vi "Read Lines From File Contrario_mio.vi"(2 "convert eol? (no:F)":bool, 3 "file path (dialog if empty)":path, 4 "number of lines (all:-1)":i32=-1, 8 "start of read offset (chars.:0)":i32, 9 "[max characters per line]  (no limit:0)":i32) -> (0 "new file path (Not A Path if cancelled)":path, 1 "line string":string, 5 "mark after read (chars.)":i32, 6 "EOF?":bool)   [LabVIEW 2010]
doc: "Reads a specified number of lines from a byte stream file beginning at a specified character offset. The VI opens the file before reading from it and closes it afterwards."
uses:
  <vilib>/Utility/error.llb/DialogType.ctl
panel:
  out "Numeric":i32
  in  "prompt":string="Choose file to read."
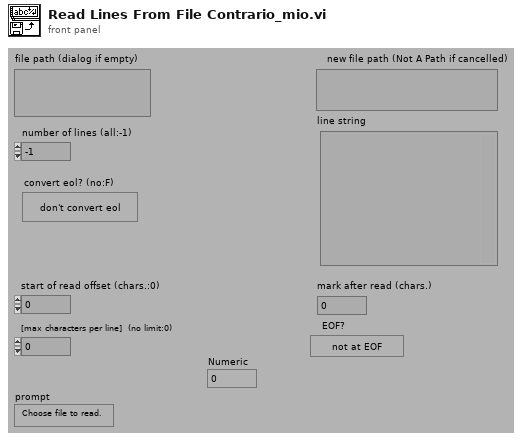
[diagram p1: front panel]
types:
  T1 = typedef "DialogType.ctl" = u16
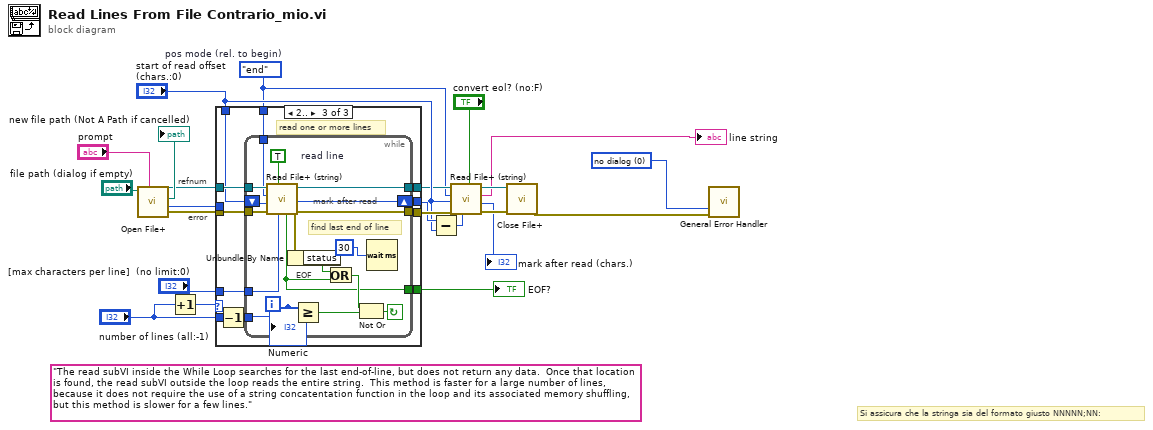
[diagram p0: block diagram]
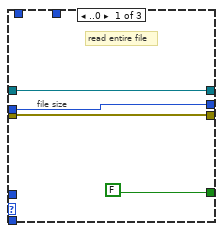
[diagram p2: hidden frame]
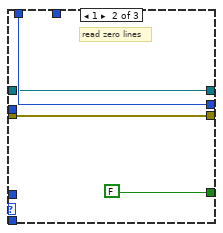
[diagram p3: hidden frame]
diagram:
  w1 = T1 0 items=["no dialog", "OK message", "continue or stop message", "OK message + warnings", "continue/stop + warnings"] ("type of dialog (OK msg:1)")
  w4 = enum16{"start", "end", "current"}."end"  # pos mode (rel. to begin)
  (unwired) "The read subVI inside the While Loop searches for the last end-of-line, but does not return any data.  Once that location is found, the read subVI outside the loop reads the entire string.  This method is faster for a large number of lines, because it does not require the use of a string concatentation function in the loop and its associated memory shuffling, but this method is slower for a few lines."
  # "Si assicura che la stringa sia del formato giusto NNNNN;NN:"
  # "error"
  # "refnum"
  n1 = call <vilib>:"Open File+.vi"("prompt"="prompt", "file path (\" \")"="file path (dialog if empty)") -> ("error out"=w11:errorcluster, "file size (bytes)"=w8:i32, "file path"=→"new file path (Not A Path if cancelled)":path, "refnum"=w10:refnum<file>)  [unwired: 6 in]
  n2 = Increment(x="number of lines (all:-1)") -> (x+1=w13:i32)
  n3 = case shown="2.." w13 {
    tunnel: [w27 w30 w42] -> w15
    tunnel: [w26 w31 w41] -> w14
    tunnel: "number of lines (all:-1)" -> [_ _ w40]
    tunnel: "[max characters per line]  (no limit:0)" -> [_ _ w39]
    tunnel: w11 -> [w27 w30 w38]
    tunnel: w10 -> [w25 w29 w37]
    tunnel: "start of read offset (chars.:0)" -> [_ w31 w36]
    tunnel: w4 -> [_ _ w35]
    tunnel: w8 -> [w26 _ _]
    tunnel: [w25 w29 w34] -> w7
    tunnel: [FALSE FALSE w33] -> w6
    frame ..0 {
      # "file size"
      # "read entire file"
    }
    frame 1 {
      # "read zero lines"
    }
    frame 2.. {
      # "read one or more lines"
      n4 = Decrement(x=w40) -> (x-1=w32:i32)
      n5 = while {
        tunnel: [w45] -> w33
        tunnel: w35 -> [w50]
        tunnel: w38 -> [w52]
        tunnel: w39 -> [w53]
        tunnel: [w48] -> w42
        tunnel: w37 -> [w55]
        tunnel: [w56] -> w34
        tunnel: w32 -> [w44]
        shift-left: w36 -> [w57]
        shift-right: [w59] -> w41
        i -> [w58]
        stop <- w51 continue-if-true
        w47 = TRUE  # read line
        # "mark after read"
        # "find last end of line"
        # "EOF"
        n6 = call <vilib>:"Read File+ (string).vi"("count"=w53, "line mode (characters:F)"=w47, "error in (no error)"=w52, "pos offset (bytes:0)"=w57, "pos mode (rel. to current:2)"=w50, "refnum"=w55) -> ("error out"=w48:errorcluster, "mark after read (bytes)"=w59:i32, "dup refnum"=w56:refnum<file>, "EOF?"=w45:bool)  [unwired: 1 in, 1 out]
        n7 = Unbundle By Name(w48) -> ("status"=w46:bool)
        n8 = Greater Or Equal?(x=w58, y=w44) -> (x >= y?=w54:bool)
        n9 = Or(x=w46, y=w45) -> (x .or. y?=w49:bool)
        n10 = Not Or(1:w54, 2:w49) -> (0:w51:bool)
        n11 = Wait (ms)(milliseconds to wait=u32 30) -> ()  [unwired: 1 out]
        "Numeric" <- w58
      }
    }
  }
  "EOF?" <- w6
  n12 = Subtract(x=w14, y="start of read offset (chars.:0)") -> (x-y=w19:i32)
  n13 = call <vilib>:"Read File+ (string).vi"("convert eol? (no:F)"="convert eol? (no:F)", "count"=w19, "error in (no error)"=w15, "pos offset (bytes:0)"="start of read offset (chars.:0)", "pos mode (rel. to current:2)"=w4, "refnum"=w7) -> ("error out"=w20:errorcluster, "mark after read (bytes)"=→"mark after read (chars.)":i32, "string"=→"line string":string, "dup refnum"=w21:refnum<file>)  [unwired: 1 in, 1 out]
  n14 = call <vilib>:"Close File+.vi"("error in (no error)"=w20, "refnum"=w21) -> ("error out"=w22:errorcluster)  [unwired: 3 in, 2 out]
  n15 = call <vilib>:"General Error Handler.vi"("type of dialog (OK msg:1)"=w1, "error in (no error)"=w22) -> ()  [unwired: 9 in, 5 out]
